vi "TCP Multiple Connections - Client - subvi - ajg.vi"(7 "Image prefix":string="IMAGE", 8 "stop 2":refnum<vi>, 10 "Port":u16=6341, 11 "Machine":string="localhost") -> (0 "warning out":errorcluster, 3 "Image Dst Out":T1)   [LabVIEW 2011]
doc: "Establishes a connection to the specified host and port and reads the date and time data sent by the Server. It first reads 4 bytes defining the length of the date & time string and then reads the data. After you click the stop button, this VI sends a single character to tell the Date Server VI to terminate the connection.\n\n<B>Note:</B> Requires the use of the Multiple Connections - Server.vi."
uses:
  <vilib>/vision/Image Controls.llb/IMAQ Image.ctl
  <vilib>/Utility/error.llb/DialogType.ctl
panel:
  in  "stop":bool
  out "error out":errorcluster
  out "# of errors":dbl
  # "Instructions:\n1. Open the Multiple Connections - Server.vi.\n2. Run the Multiple Connections - Server.vi first.\n3. Run the Client VIs second.\n4. Stop this VI and restart it to notice the # of Connections on the Server VI change.\n5. Stop the Server VI.  This VI will stop when it times out."
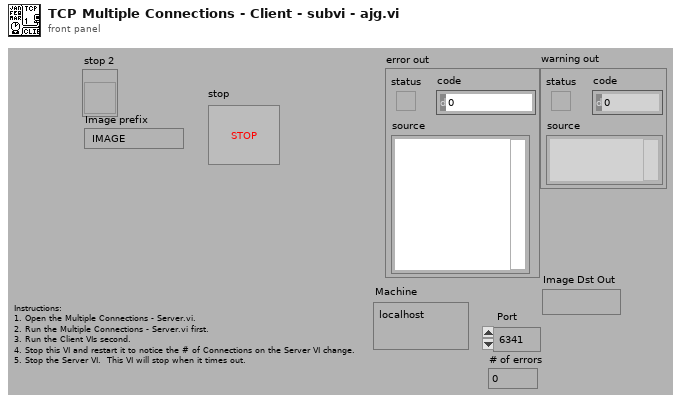
[diagram p1: front panel]
types:
  T1 = typedef "IMAQ Image.ctl" = refnum<image>
  T2 = typedef "DialogType.ctl" = u16
  T3 = typedef "Image Type" = u32
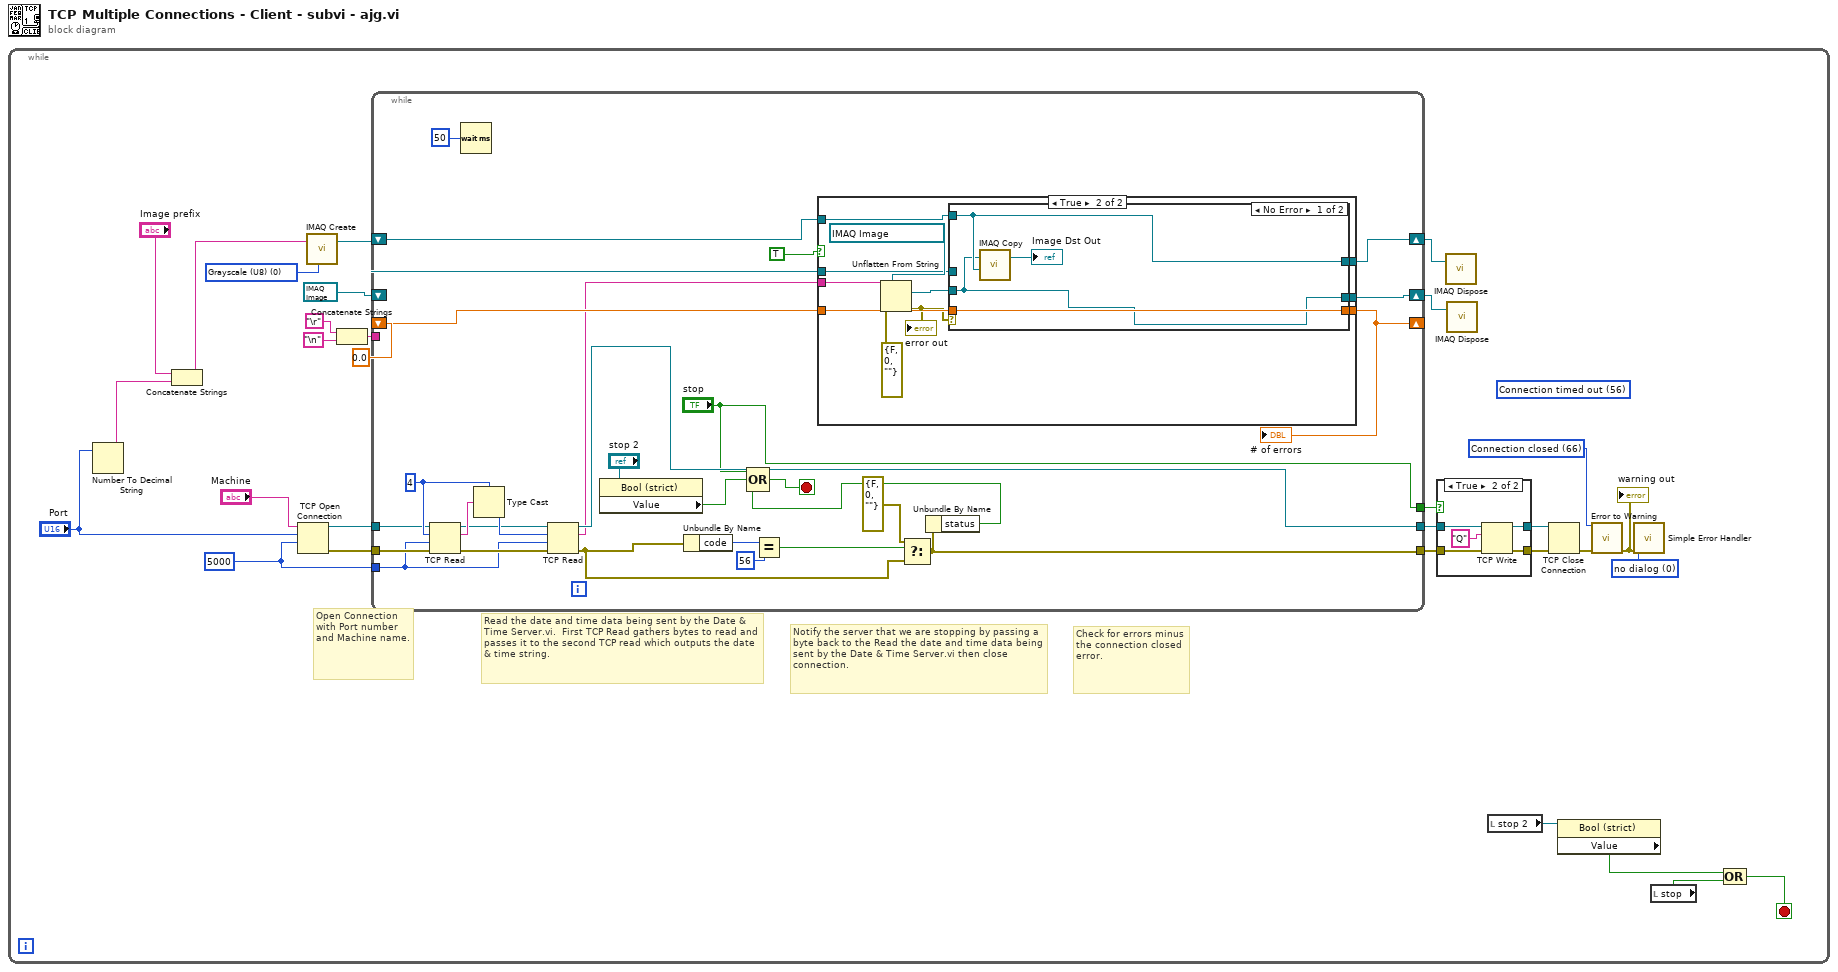
[diagram p0: block diagram]
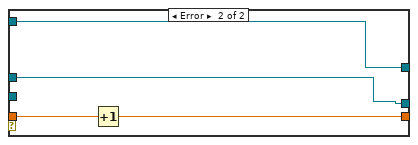
[diagram p3: hidden frame]
diagram:
  n1 = while {
    stop <- w1 stop-if-true
    (unwired) 56 items=["No Error", "Argument Error", "Memory Full", "Out of Zone", "End of File", "File Already Open", "Generic File IO Error", "File Not Found", "File Permission Error", "Disk Full", "Duplicate Path", "Too Many Files Open", "Not Enabled", "Resource File Not Found", "Cannot Add Resource", "Resource Not Found", "Image Not Found", "Image Memory Error", "Pen Does Not Exist", "Config Bad Type", "Config Token Not Found", "Config Parse Error", "Config Memory Error", "Bad External Code Format", "Bad External Code Offset", "External Code Not Present", "Null Window", "Destroy Window Mixup", "Null Menu", "Print Aborted", "Bad Print Record", "Print Driver Error", "Windows Error During Print", "Memory Error During Print", "Print Dialog Error", "Generic Print Error", "Invalid Device Refnum", "Device Not Found", "Device Parameter Error", "Device Unit Error", "Can't Open Device", "Device Call Aborted", "Generic Error", "Cancelled By User", "Object ID Too Low", "Object ID Too High", "Object Not In Heap", "Unknown Heap", "Bad DefProc ID", "DefProc Not In Table", "Message Out Of Range", "Null Method", "Unknown Message", "Manager Call Not Supported", "Bad address", "Connection In progress", "Connection timed out", "Connection is already in progress", "Network attribute not supported", "Network error", "Address in use", "System out of memory", "Connection aborted", "Connection refused", "Connection is not connected", "Connection is already connected", "Connection closed", "Initialize error (interapplication manager)", "Bad occurrence", "Wait on unbound occurrence handler", "Occurrence queue overflow", "Bad path", "Semaphore not signaled", "Unrecognized type (interapplication manager)"] ("1st Error to Convert")
    w5 = 5000 ("timeout ms (25000)")
    w6 = T2 0 items=["no dialog", "OK message", "continue or stop message", "OK message + warnings", "continue/stop + warnings"] ("type of dialog (OK msg:1)")
    w17 = T3 0 items=["Grayscale (U8)", "Grayscale (I16)", "Grayscale (SGL)", "Complex (CSG)", "RGB (U32)", "HSL (U32)", "RGB (U64)", "Grayscale (U16)"] ("Image Type")
    w22 = 66 items=["No Error", "Argument Error", "Memory Full", "Out of Zone", "End of File", "File Already Open", "Generic File IO Error", "File Not Found", "File Permission Error", "Disk Full", "Duplicate Path", "Too Many Files Open", "Not Enabled", "Resource File Not Found", "Cannot Add Resource", "Resource Not Found", "Image Not Found", "Image Memory Error", "Pen Does Not Exist", "Config Bad Type", "Config Token Not Found", "Config Parse Error", "Config Memory Error", "Bad External Code Format", "Bad External Code Offset", "External Code Not Present", "Null Window", "Destroy Window Mixup", "Null Menu", "Print Aborted", "Bad Print Record", "Print Driver Error", "Windows Error During Print", "Memory Error During Print", "Print Dialog Error", "Generic Print Error", "Invalid Device Refnum", "Device Not Found", "Device Parameter Error", "Device Unit Error", "Can't Open Device", "Device Call Aborted", "Generic Error", "Cancelled By User", "Object ID Too Low", "Object ID Too High", "Object Not In Heap", "Unknown Heap", "Bad DefProc ID", "DefProc Not In Table", "Message Out Of Range", "Null Method", "Unknown Message", "Manager Call Not Supported", "Bad address", "Connection In progress", "Connection timed out", "Connection is already in progress", "Network attribute not supported", "Network error", "Address in use", "System out of memory", "Connection aborted", "Connection refused", "Connection is not connected", "Connection is already connected", "Connection closed", "Initialize error (interapplication manager)", "Bad occurrence", "Wait on unbound occurrence handler", "Occurrence queue overflow", "Bad path", "Semaphore not signaled", "Unrecognized type (interapplication manager)"] ("1st Error to Convert")
    # "Check for errors minus the connection closed error."
    # "Notify the server that we are stopping by passing a byte back to the Read the date and time data being sent by the Date & Time Server.vi then close connection."
    # "Read the date and time data being sent by the Date & Time Server.vi.  First TCP Read gathers bytes to read and passes it to the second TCP read which outputs the date & time string."
    # "Open Connection with Port number and Machine name."
    n2 = Number To Decimal String(number="Port") -> (decimal integer string=w8:string)  [unwired: 1 in]
    n3 = Concatenate Strings("Image prefix", w8) -> (w10:string)
    n4 = TCP Open Connection(address="Machine", remote port or service name="Port", timeout ms (60000)=w5) -> (connection ID=w30:refnum<k5>, error out=w29:errorcluster)  [unwired: 1 in, 1 out]
    n5 = call "IMAQ Create"("Image Name"=w10, "Image Type"=w17) -> ("New Image"=w16:T1)  [unwired: 3 in, 1 out]
    n6 = Concatenate Strings("\r", "\n") -> (w19:string)
    n7 = while {
      tunnel: [w59] -> w28
      tunnel: [w32] -> w26
      tunnel: w29 -> [w50]
      tunnel: w30 -> [w49]
      tunnel: w19 -> [_]
      shift-right: [w56] -> _
      shift-left: 0.0 -> [w55]
      shift-right: [w44] -> w15
      shift-left: w16 -> [w45]
      shift-right: [w43] -> w13
      shift-left: T1 refnum ("New Image") -> [w42]
      tunnel: ["stop"] -> w9
      tunnel: w5 -> [w33]
      stop <- w58 stop-if-true
      w54 = 4
      n8 = TCP Read(connection ID=w49, bytes to read=w54, error in (no error)=w50, 9:w33) -> (connection ID out=w48:refnum<k5>, data out=w53:string, error out=w51:errorcluster)  [unwired: 1 in]
      n9 = Wait (ms)(milliseconds to wait=u32 50) -> ()  [unwired: 1 out]
      n10 = Type Cast(type=w54, x=w53) -> (*(type *) &x=w52:i32)
      n11 = TCP Read(connection ID=w48, bytes to read=w52, error in (no error)=w51, 9:w33) -> (connection ID out=w59:refnum<k5>, data out=w47:string, error out=w35:errorcluster)  [unwired: 1 out]
      n12 = property class="Bool (strict)"(reference="stop 2") -> ("Value"=w40:bool)  [unwired: 1 in, 2 out]
      n13 = Unbundle By Name(w35) -> ("code"=w38:i32)
      n14 = Equal?(x=w38, y=56) -> (x = y?=w36:bool)
      n15 = case shown="True" TRUE {
        tunnel: w47 -> [_ w68]
        tunnel: [w62 w72] -> w56
        tunnel: w55 -> [w62 w71]
        tunnel: [w61 w66] -> w44
        tunnel: w45 -> [w61 w65]
        tunnel: [w60 w64] -> w43
        tunnel: w42 -> [w60 w63]
        frame False {
        }
        frame True {
          n16 = Unflatten From String(type=T1 refnum ("New Image"), binary string=w68, error in (no error)=errorcluster {"status"=FALSE, "code"=0, "source"=""}) -> (value=w73:T1, error out=w70:errorcluster)  [unwired: 3 out]
          "error out" <- w70
          n17 = case shown="No Error" w70 {
            tunnel: w73 -> [w74 _]
            tunnel: [w77 w80] -> w72
            tunnel: w71 -> [w77 w81]
            tunnel: [w76 w79] -> w66
            tunnel: w65 -> [w76 w79]
            tunnel: [w74 w78] -> w64
            tunnel: w63 -> [_ w78]
            frame No Error {
              n18 = call "IMAQ Copy"("Image Dst"=w76, "Image Src"=w74) -> ("Image Dst Out"=→"Image Dst Out":T1)  [unwired: 4 in, 1 out]
            }
            frame Error {
              n19 = Increment(x=w81) -> (x+1=w80:dbl)
            }
          }
        }
      }
      "# of errors" <- w56
      n20 = Select(t=errorcluster {"status"=FALSE, "code"=0, "source"=""}, s=w36, f=w35) -> (s? t:f=w32:errorcluster)
      n21 = Unbundle By Name(w32) -> ("status"=w31:bool)
      n22 = Compound Arithmetic op=OR("stop", w40, w31) -> (w58:bool)
    }
    n23 = case shown="True" w9 {
      tunnel: w28 -> [w83 w88]
      tunnel: [w83 w86] -> w27
      tunnel: w26 -> [w82 w87]
      tunnel: [w82 w85] -> w25
      frame False {
      }
      frame True {
        n24 = TCP Write(connection ID=w88, data in="Q", error in (no error)=w87) -> (connection ID out=w86:refnum<k5>, error out=w85:errorcluster)  [unwired: 2 out]
      }
    }
    n25 = call "IMAQ Dispose"("Image"=w15) -> ()  [unwired: 5 in, 1 out]
    n26 = call "IMAQ Dispose"("Image"=w13) -> ()  [unwired: 5 in, 1 out]
    n27 = local read "stop 2"() -> (w4:refnum<vi>)
    n28 = TCP Close Connection(connection ID=w27, error in (no error)=w25) -> (error out=w24:errorcluster)  [unwired: 2 out]
    n29 = property class="Bool (strict)"(reference=w4) -> ("Value"=w3:bool)  [unwired: 1 in, 2 out]
    n30 = call <vilib>:"Error to Warning.vi"("1st Error to Convert"=w22, "error in"=w24) -> ("warning out"=w23:errorcluster)  [unwired: 3 in, 10 out]
    "warning out" <- w23
    n31 = call <vilib>:"Simple Error Handler.vi"("type of dialog (OK msg:1)"=w6, "error in (no error)"=w23) -> ()  [unwired: 8 out]
    n32 = local read "stop"() -> (w2:bool)
    n33 = Compound Arithmetic op=OR(w3, w2) -> (w1:bool)
  }
